vi "Array_3.vi"() -> ()   [LabVIEW 2018]
panel:
  out "Intensity Chart":dbl[][](graph)
  in  "Строки":i32
  in  "Столбцы":i32
  out "Массив":dbl[][](array[numeric])
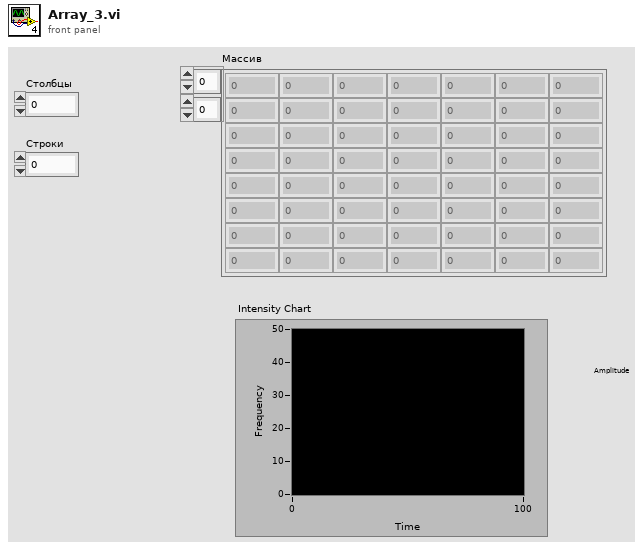
[diagram p1: front panel]
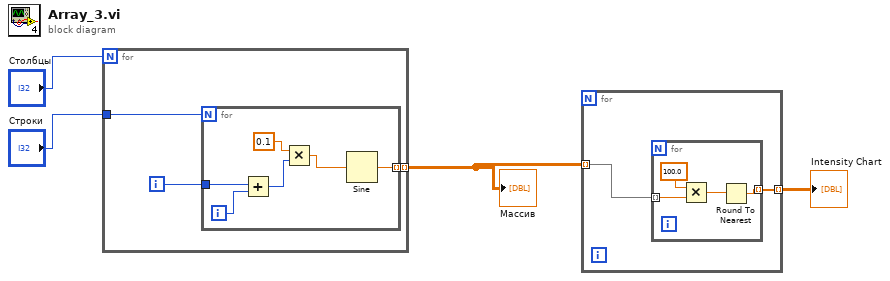
[diagram p0: block diagram]
diagram:
  n1 = for {
    N: "Столбцы" -> [_]
    tunnel: "Строки" -> [w6]
    tunnel: [w5] -> w2 mode=indexing
    i -> [w7]
    n2 = for {
      N: w6 -> [_]
      tunnel: w7 -> [w12]
      tunnel: [w8] -> w5 mode=indexing
      i -> [w13]
      n3 = Add(x=w12, y=w13) -> (x+y=w10:i32)
      n4 = Multiply(x=0.1, y=w10) -> (x*y=w9:dbl)
      n5 = Sine(x=w9) -> (sin(x)=w8:dbl)
    }
  }
  "Массив" <- w2
  n6 = for {
    tunnel: w2 -> [w15] mode=indexing
    tunnel: [w14] -> w1 mode=indexing
    n7 = for {
      tunnel: w15 -> [w18] mode=indexing
      tunnel: [w16] -> w14 mode=indexing
      n8 = Multiply(x=100.0, y=w18) -> (x*y=w17:dbl)
      n9 = Round To Nearest(number=w17) -> (nearest integer value=w16:dbl)
    }
  }
  "Intensity Chart" <- w1
